vi "Switch Sides.vi"(10 "Lado":enum16{"Esquerdo", "Direito"}(ring) caption="Enum", 11 "Detection Frame":T1={"our_robots"=[], "enemy_robots"=[], "balls"=[], "geometry"={"field_length"=0, "field_width"=0, "goal_width"=0, "goal_depth"=0, "center_circle_radius"=0, "defense_width"=0, "defense_depth"=0, "free_kick_from_defense_dist"=0, "penalty_spot_from_field_line_dist"=0, "penalty_line_from_spot_dist"=0, "half_moon_depth"=0, "half_moon_width"=0}, "IA Judge"={"stage"="", "command"="", "our_goalie_id"=0.0, "enemy_goalie_id"=0.0, "command enum"=enum."Halt", "Time"=enum."Azul"}, "Received Timestamp"=timestamp(0 s since 1904-01-01), "Events"={"Touch"=FALSE, "Ball out"=FALSE, "id touch"=0.0, "Ball out of \nVision"=FALSE, "Ball inside \nGoalie area"=FALSE, "Robot not responding"=FALSE, "Robots responding status"=[1.0, 1.0, 1.0, 1.0, 1.0, 1.0], "Enemy Ball \nPossession"=FALSE, "Pass State"=FALSE, "id end of pass"=0.0, "Kick"=FALSE, "Id ini Possession"=0.0, "Ball Possesion"=FALSE, "Id Possesion"=0.0}}) -> (3 "Detection Frame 2":T1={"our_robots"=[], "enemy_robots"=[], "balls"=[], "geometry"={"field_length"=0, "field_width"=0, "goal_width"=0, "goal_depth"=0, "center_circle_radius"=0, "defense_width"=0, "defense_depth"=0, "free_kick_from_defense_dist"=0, "penalty_spot_from_field_line_dist"=0, "penalty_line_from_spot_dist"=0, "half_moon_depth"=0, "half_moon_width"=0}, "IA Judge"={"stage"="", "command"="", "our_goalie_id"=0.0, "enemy_goalie_id"=0.0, "command enum"=enum."Halt", "Time"=enum."Azul"}, "Received Timestamp"=timestamp(0 s since 1904-01-01), "Events"={"Touch"=FALSE, "Ball out"=FALSE, "id touch"=0.0, "Ball out of \nVision"=FALSE, "Ball inside \nGoalie area"=FALSE, "Robot not responding"=FALSE, "Robots responding status"=[1.0, 1.0, 1.0, 1.0, 1.0, 1.0], "Enemy Ball \nPossession"=FALSE, "Pass State"=FALSE, "id end of pass"=0.0, "Kick"=FALSE, "Id ini Possession"=0.0, "Ball Possesion"=FALSE, "Id Possesion"=0.0}})   [LabVIEW 2017]
uses:
  AI Input.ctl
  AI Robot.ctl
  Intel/Functions Enum.ctl
  Intel/AttackerStates.ctl
  Path Planning/RRT/PathDests.ctl
  Path Planning/RRT/PathDest.ctl
  AI Ball.ctl
  Field Size.ctl
  AI Judge.ctl
  Intel/Command Enum.ctl
  Util/Events/Events.ctl
  <vilib>/Analysis/coordinate.llb/Wrap Angle (scalar).vi
  <vilib>/Analysis/NI_AAL_Angle.lvlib
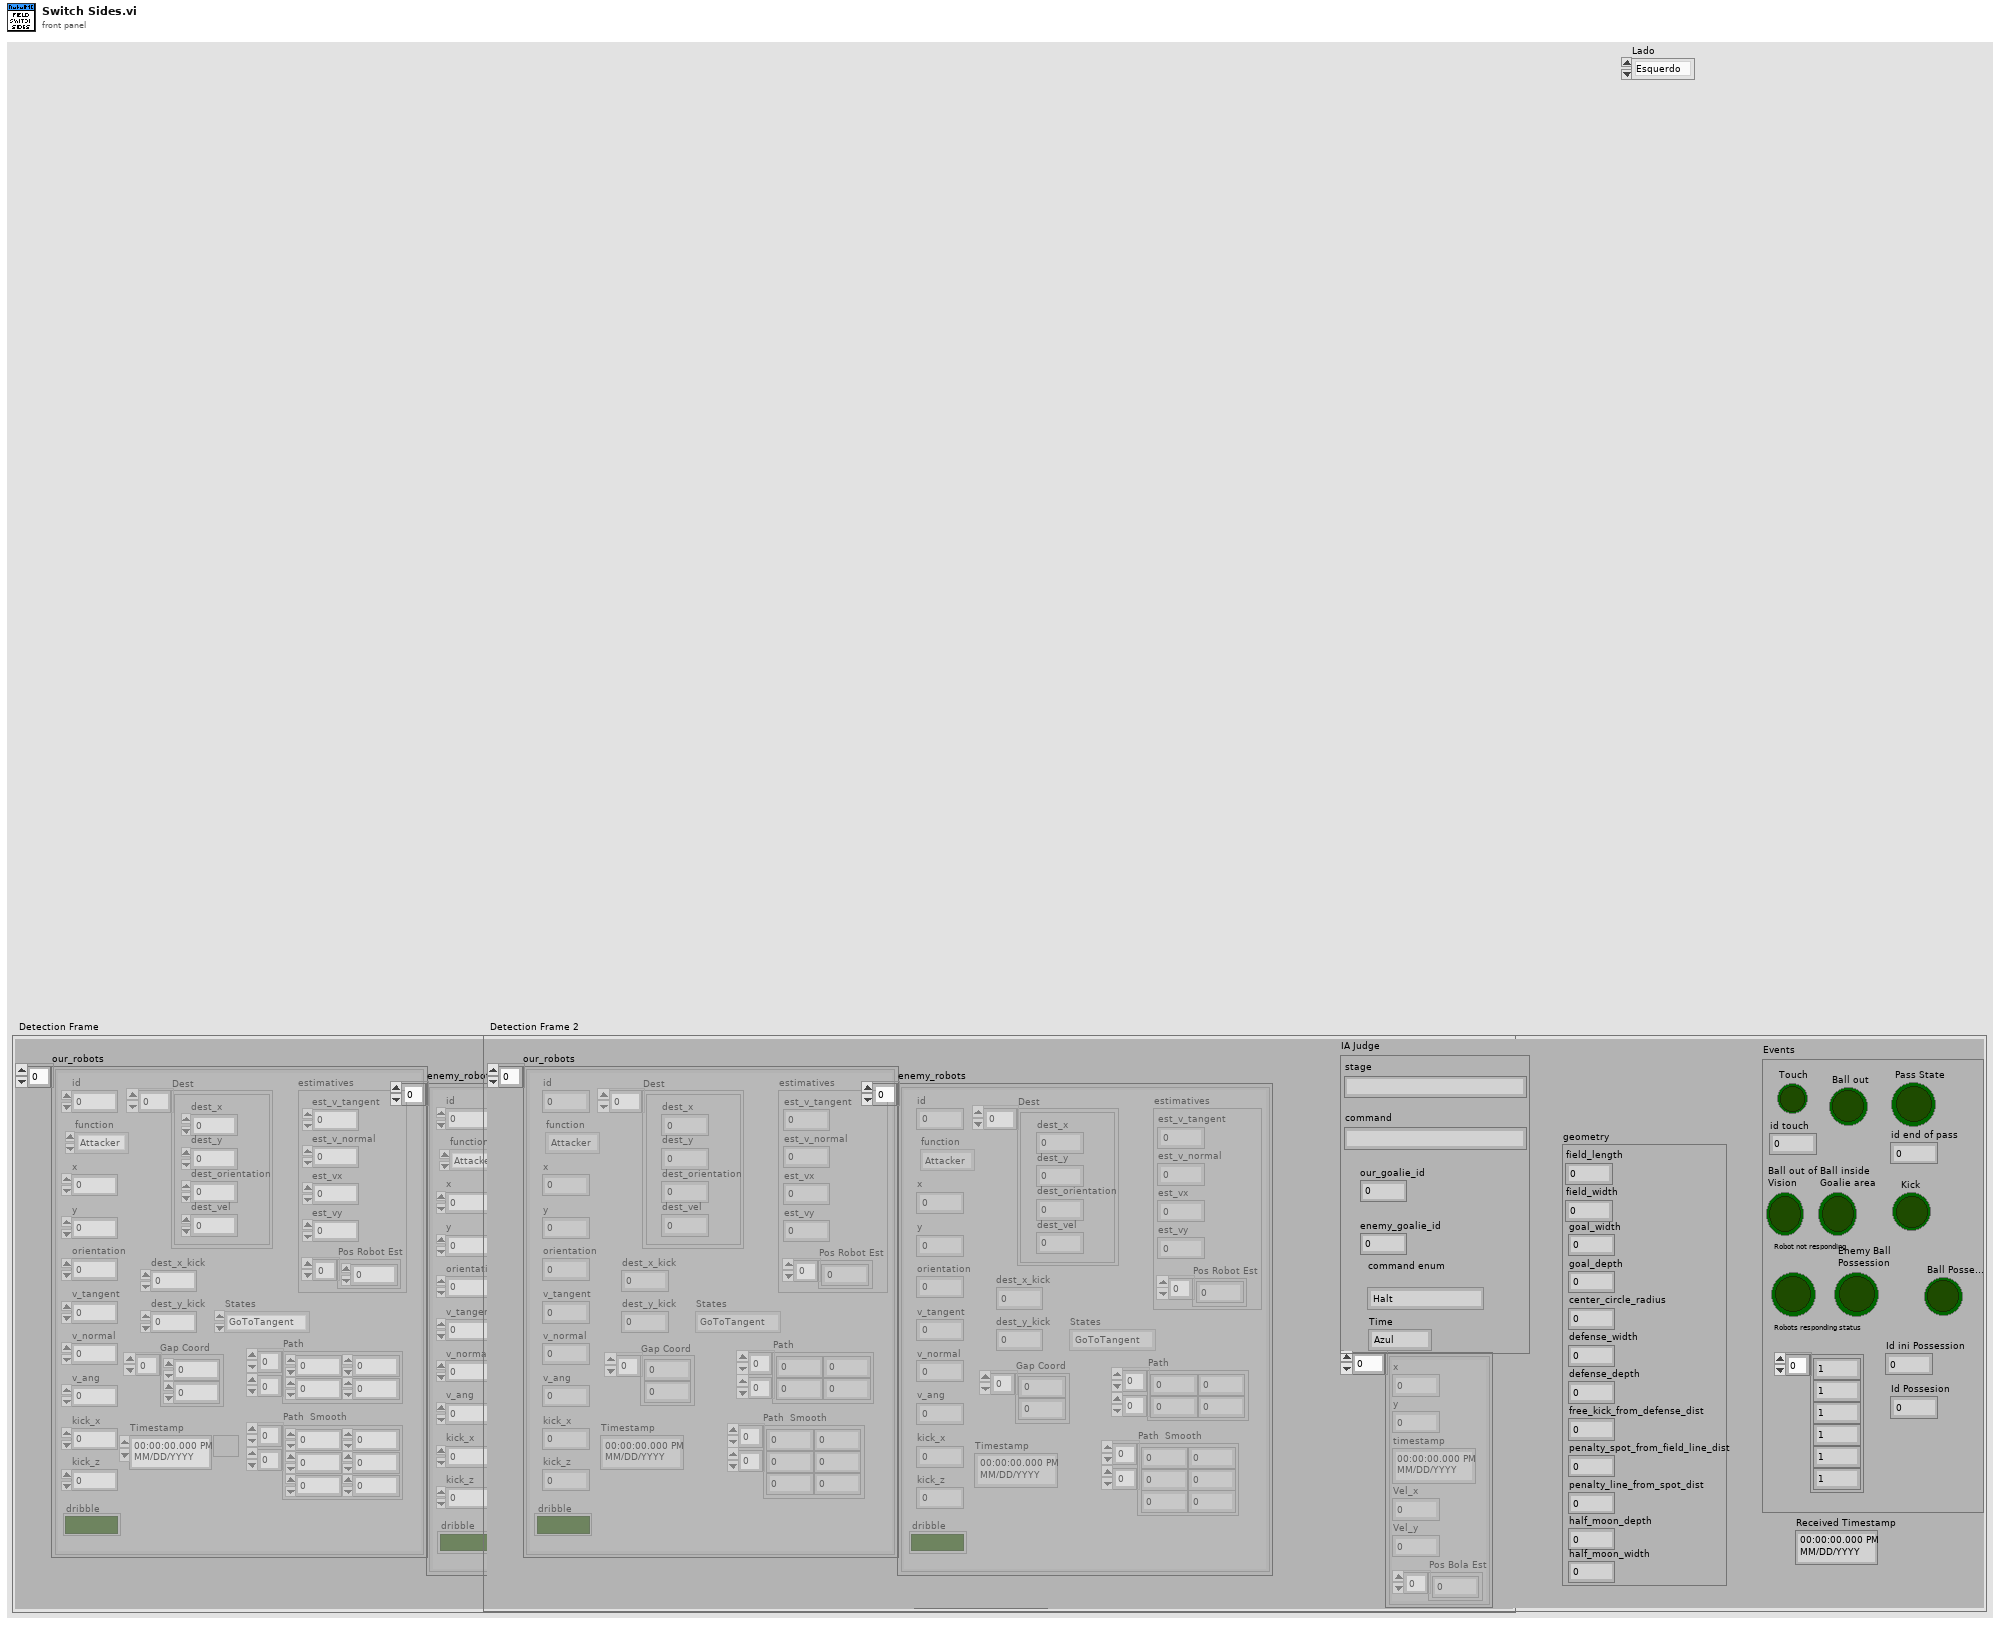
[diagram p1: front panel]
types:
  T1 = typedef "AI Input.ctl" = cluster{"our_robots":T2[], "enemy_robots":T2[], "balls":T7[], "geometry":T8, "IA Judge":T9, "Received Timestamp":timestamp, "Events":T11}
  T2 = typedef "AI Robot.ctl" = cluster{"id":u32, "function":T3, "x":dbl, "y":dbl, "orientation":dbl, "v_tangent":dbl, "v_normal":dbl, "v_ang":dbl, "kick_x":dbl, "kick_z":dbl, "dribble":bool, "Timestamp":timestamp, "estimatives":cluster{"est_v_tangent":dbl, "est_v_normal":dbl, "est_vx":dbl, "est_vy":dbl, "Pos Robot Est":dbl[]}, "dest_x_kick":dbl, "dest_y_kick":dbl, "Gap Coord":dbl[], "States":T4, "Path ":dbl[][], "Path  Smooth":dbl[][], "Dest":T5}
  T3 = typedef "Functions Enum.ctl" = enum16{"Attacker", "Goalie", "Defender", "Striker", "Goto 0", "Dummy", "Kicker", "ZigZag"}
  T4 = typedef "AttackerStates.ctl" = enum16{"Pass", "GoToTangent", "BallGetting", "GoToKick", ""}
  T5 = typedef "PathDests.ctl" = T6[]
  T6 = typedef "PathDest.ctl" = cluster{"dest_x":dbl, "dest_y":dbl, "dest_orientation":dbl, "dest_vel":dbl}
  T7 = typedef "AI Ball.ctl" = cluster{"x":dbl, "y":dbl, "timestamp":timestamp, "Vel_x":dbl, "Vel_y":dbl, "Pos Bola Est":dbl[]}
  T8 = typedef "Field Size.ctl" = cluster{"field_length":u32, "field_width":u32, "goal_width":u32, "goal_depth":u32, "center_circle_radius":u32, "defense_width":u32, "defense_depth":u32, "free_kick_from_defense_dist":u32, "penalty_spot_from_field_line_dist":u32, "penalty_line_from_spot_dist":u32, "half_moon_depth":u32, "half_moon_width":u32}
  T9 = typedef "AI Judge.ctl" = cluster{"stage":string, "command":string, "our_goalie_id":dbl, "enemy_goalie_id":dbl, "command enum":T10, "Time":enum16{"Azul", "Amarelo"}}
  T10 = typedef "Command Enum.ctl" = enum16{"Halt", "Stop", "Force Start", "PKA Normal Start", "Prepare Kickoff Ally", "PKE Normal Start", "Prepare Kickoff Enemy", "Prepare Penalty Ally", "PPA Normal Start", "Prepare Penalty Enemy", "PPE Normal Start", "Direct Free Enemy", "Direct Free Ally", "Indirect Free Enemy", "Indirect Free Ally", "Timeout Enemy", "Timeout Ally", "Goal Enemy", "Goal Ally", "Ball Placement Enemy", "Ball Placement Ally", "Normal Half Time", "Extra Time Break", "Extra Half Time", "None", "Post Game"}
  T11 = typedef "Events.ctl" = cluster{"Touch":bool, "Ball out":bool, "id touch":dbl, "Ball out of \nVision":bool, "Ball inside \nGoalie area":bool, "Robot not responding":bool, "Robots responding status":dbl[], "Enemy Ball \nPossession":bool, "Pass State":bool, "id end of pass":dbl, "Kick":bool, "Id ini Possession":dbl, "Ball Possesion":bool, "Id Possesion":dbl}
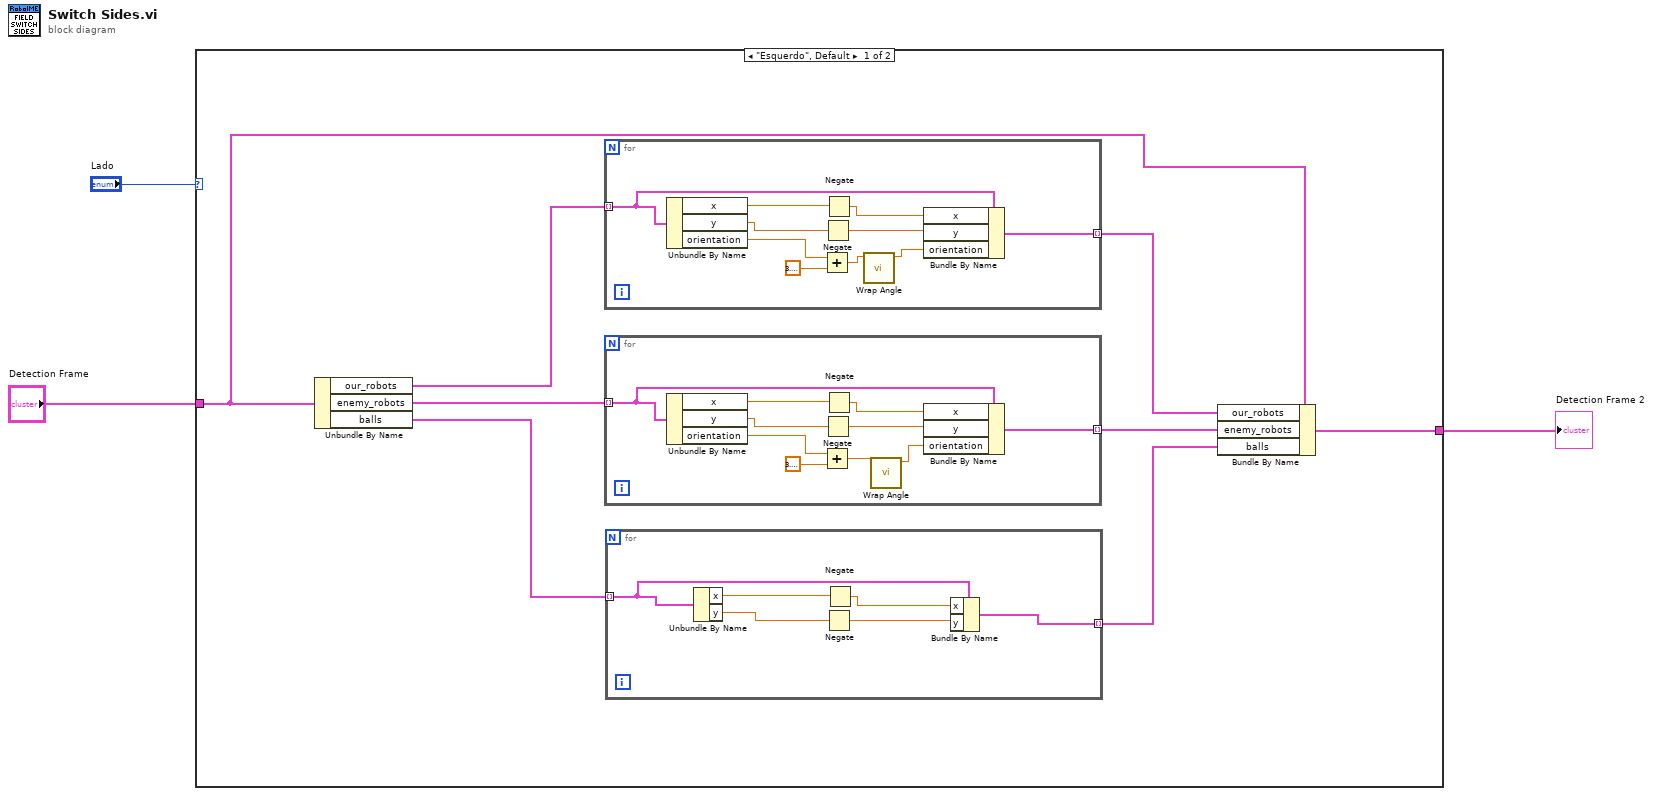
[diagram p0: block diagram]
diagram:
  n1 = case shown="\"Esquerdo\", Default" "Lado" {
    tunnel: "Detection Frame" -> [w5 w38]
    tunnel: [w4 w38] -> w1
    frame "Esquerdo", Default {
      n2 = Unbundle By Name(w5) -> ("our_robots"=w11:T2[], "enemy_robots"=w9:T2[], "balls"=w7:T7[])
      n3 = for {
        tunnel: w11 -> [w33] mode=indexing
        tunnel: [w30] -> w10 mode=indexing
        n4 = Unbundle By Name(w33) -> ("x"=w37:dbl, "y"=w36:dbl, "orientation"=w34:dbl)
        n5 = Add(x=w34, y=3.141592653589793) -> (x+y=w29:dbl)
        n6 = Negate(x=w36) -> (-x=w31:dbl)
        n7 = Negate(x=w37) -> (-x=w32:dbl)
        n8 = call-poly <vilib>:"Wrap Angle.vi"("angle in"=w29) -> ("angle out"=w28:dbl)  [unwired: 9 in, 1 out]
        n9 = Bundle By Name(cluster=w33, "x"=w32, "y"=w31, "orientation"=w28) -> (w30:T2)
      }
      n10 = for {
        tunnel: w9 -> [w17] mode=indexing
        tunnel: [w14] -> w8 mode=indexing
        n11 = Unbundle By Name(w17) -> ("x"=w21:dbl, "y"=w20:dbl, "orientation"=w18:dbl)
        n12 = Add(x=w18, y=3.141592653589793) -> (x+y=w13:dbl)
        n13 = Negate(x=w20) -> (-x=w15:dbl)
        n14 = Negate(x=w21) -> (-x=w16:dbl)
        n15 = call-poly <vilib>:"Wrap Angle.vi"("angle in"=w13) -> ("angle out"=w12:dbl)  [unwired: 9 in, 1 out]
        n16 = Bundle By Name(cluster=w17, "x"=w16, "y"=w15, "orientation"=w12) -> (w14:T2)
      }
      n17 = for {
        tunnel: w7 -> [w25] mode=indexing
        tunnel: [w22] -> w6 mode=indexing
        n18 = Unbundle By Name(w25) -> ("x"=w27:dbl, "y"=w26:dbl)
        n19 = Negate(x=w26) -> (-x=w23:dbl)
        n20 = Negate(x=w27) -> (-x=w24:dbl)
        n21 = Bundle By Name(cluster=w25, "x"=w24, "y"=w23) -> (w22:T7)
      }
      n22 = Bundle By Name(cluster=w5, "our_robots"=w10, "enemy_robots"=w8, "balls"=w6) -> (w4:T1)
    }
    frame "Direito" {
    }
  }
  "Detection Frame 2" <- w1
